vi "CommonVIs_StringToConfigData.vi"(0 "string input":string, 1 "RemoveStartAnmdEndQuotes(YES)":bool=TRUE) -> (14 "section names":string[](array[string]), 15 "data":T1[](array[typedef]))   [LabVIEW 2014]
uses:
  <vilib>/Utility/config.llb/Config Data Section.ctl
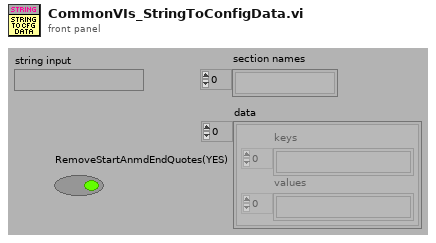
[diagram p1: front panel]
types:
  T1 = typedef "Config Data Section.ctl" = cluster{"keys":string[], "values":string[]}
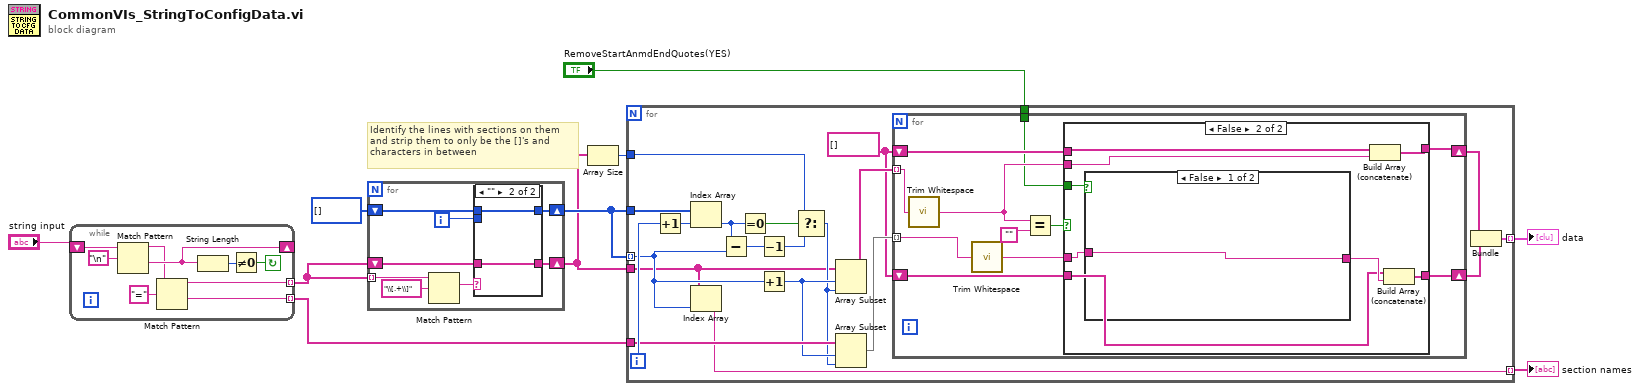
[diagram p0: block diagram]
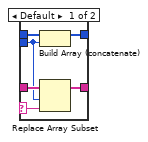
[diagram p2: hidden frame]
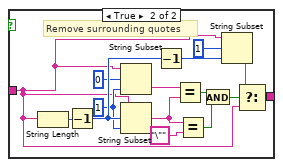
[diagram p4: hidden frame]
diagram:
  # "Identify the lines with sections on them\nand strip them to only be the []'s and \ncharacters in between"
  n1 = while {
    shift-left: "string input" -> [w14]
    shift-right: [w12] -> _
    tunnel: [w16] -> w5 mode=indexing
    tunnel: [w17] -> w3 mode=indexing
    stop <- w15 continue-if-true
    n2 = Match Pattern(string=w14, regular expression="\n") -> (before substring=w11:string, after substring=w12:string)  [unwired: 3 out]
    n3 = Match Pattern(string=w11, regular expression="=") -> (before substring=w17:string, after substring=w16:string)  [unwired: 3 out]
    n4 = String Length(string=w12) -> (length=w13:i32)
    n5 = Not Equal To 0?(x=w13) -> (x != 0?=w15:bool)
  }
  n6 = for {
    tunnel: w3 -> [w27] mode=indexing
    shift-right: [w24] -> w9
    shift-left: i32[] [] -> [w23]
    shift-right: [w21] -> w4
    shift-left: w3 -> [w20]
    i -> [w25]
    n7 = Match Pattern(string=w27, regular expression="\\[.+\\]") -> (match substring=w22:string)  [unwired: 4 out]
    n8 = case shown="\"\"" w22 {
      selector: w22 -> [w29 _]
      tunnel: w25 -> [w28 _]
      tunnel: [w32 w35] -> w24
      tunnel: w23 -> [w33 w35]
      tunnel: [w30 w34] -> w21
      tunnel: w20 -> [w31 w34]
      frame Default {
        n9 = Build Array (concatenate)(w33, w28) -> (w32:i32[])
        n10 = Replace Array Subset(array=w31, new element=w29, index=w28) -> (w30:string[])
      }
      frame "" {
      }
    }
  }
  n11 = Array Size(array=w4) -> (size(s)=w6:i32)
  n12 = for {
    tunnel: w9 -> [w51] mode=indexing
    tunnel: w4 -> [w39]
    tunnel: w5 -> [w53]
    tunnel: w9 -> [w56]
    tunnel: [w49] -> w2 mode=indexing
    tunnel: [w44] -> w7 mode=indexing
    tunnel: w6 -> [w38]
    tunnel: "RemoveStartAnmdEndQuotes(YES)" -> [w36]
    i -> [w54]
    w37 = string[] []
    n13 = Increment(x=w54) -> (x+1=w55:i32)
    n14 = Index Array(array=w56, index=w55) -> (element=w48:i32)
    n15 = Index Array(array=w39, index=w51) -> (element=w44:string)
    n16 = Subtract(x=w48, y=w51) -> (x-y=w50:i32)
    n17 = Equal To 0?(x=w48) -> (x = 0?=w47:bool)
    n18 = Decrement(x=w50) -> (x-1=w46:i32)
    n19 = Increment(x=w51) -> (x+1=w52:i32)
    n20 = Select(t=w38, s=w47, f=w46) -> (s? t:f=w45:i32)
    n21 = Array Subset(array=w39, index=w52, length=w45) -> (w43:string[])
    n22 = Array Subset(array=w53, index=w52, length=w45) -> (w42:string[])
    n23 = for {
      tunnel: w43 -> [w62] mode=indexing
      tunnel: w42 -> [w60] mode=indexing
      shift-right: [w65] -> w40
      shift-left: w37 -> [w66]
      shift-right: [w63] -> w41
      shift-left: w37 -> [w64]
      tunnel: w36 -> [w57]
      n24 = call <vilib>:"Trim Whitespace.vi"("string"=w62) -> ("trimmed string"=w61:string)  [unwired: 1 in]
      n25 = call <vilib>:"Trim Whitespace.vi"("string"=w60) -> ("trimmed string"=w59:string)  [unwired: 1 in]
      n26 = Equal?(x=w61, y="") -> (x = y?=w58:bool)
      n27 = case shown="False" w58 {
        tunnel: w59 -> [_ w77]
        tunnel: w66 -> [w69 w75]
        tunnel: [w69 w76] -> w65
        tunnel: w61 -> [_ w74]
        tunnel: [w68 w73] -> w63
        tunnel: w64 -> [w68 w71]
        tunnel: w57 -> [_ w70]
        frame True {
        }
        frame False {
          n28 = case shown="False" w70 {
            tunnel: w77 -> [w78 w80]
            tunnel: [w78 w79] -> w72
            frame False {
            }
            frame True {
              w82 = 1 ("length")
              # "Remove surrounding quotes"
              n29 = String Length(string=w80) -> (length=w84:i32)
              n30 = Decrement(x=w84) -> (x-1=w91:i32)
              n31 = String Subset(string=w80, offset (0)=0, length (rest)=w82) -> (substring=w86:string)
              n32 = String Subset(string=w80, offset (0)=w91, length (rest)=w82) -> (substring=w81:string)
              n33 = Decrement(x=w91) -> (x-1=w92:i32)
              n34 = Equal?(x=w86, y=w81) -> (x = y?=w87:bool)
              n35 = Equal?(x=w81, y="\"") -> (x = y?=w89:bool)
              n36 = And(x=w87, y=w89) -> (x .and. y?=w85:bool)
              n37 = String Subset(string=w80, offset (0)=1, length (rest)=w92) -> (substring=w93:string)
              n38 = Select(t=w93, s=w85, f=w80) -> (s? t:f=w79:string)
            }
          }
          n39 = Build Array (concatenate)(w75, w74) -> (w76:string[])
          n40 = Build Array (concatenate)(w71, w72) -> (w73:string[])
        }
      }
    }
    n41 = Bundle(w40, w41) -> (w49:cluster{string[], string[]})  [unwired: 1 out]
  }
  "data" <- w2
  "section names" <- w7
